vi "close_com.vi"(8 "error in (no error)":errorcluster) -> (0 "error out":errorcluster)   [LabVIEW 2016, in "BT-Android_interface.lvlib"]
uses:
  BT-Android_interface.lvlib
  mode.ctl
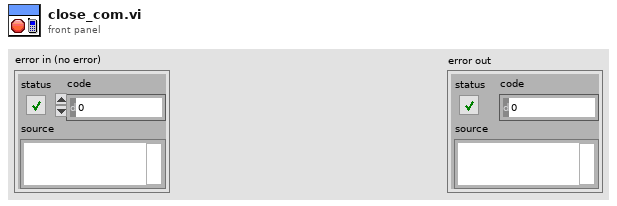
[diagram p1: front panel]
types:
  T1 = typedef "BT-Android_interface.lvlib/mode.ctl" = enum16{"init", "broadcast_data", "receive_data", "close"}
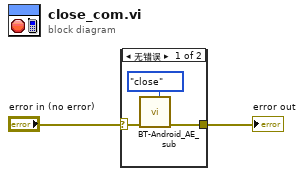
[diagram p0: block diagram]
diagram:
  n1 = case shown="无错误" "error in (no error)" {
    selector: "error in (no error)" -> [w5 w6]
    tunnel: [w4 w6] -> w1
    frame No Error {
      n2 = call "BT-Android_AE_sub.vi"("mode"=mode."close", "error in (no error)"=w5) -> ("error IO"=w4:errorcluster)  [unwired: 8 in, 1 out]
    }
    frame Error {
    }
  }
  "error out" <- w1
